vi "Array Test.vi"() -> ()   [LabVIEW 2016]
uses:
  Source/Shared Memory/Controls/file mode.ctl
  <vilib>/NI/Memory Manager/Classes/Pointer/Pointer.lvclass/Pointer.ctl
  <vilib>/NI/Memory Manager/Classes/Pointer/Write (1D DBL).vi
  <vilib>/NI/Memory Manager/Classes/Pointer/Read (1D DBL).vi
  <vilib>/NI/Memory Manager/Classes/Pointer/Write (1D Bool).vi
  <vilib>/NI/Memory Manager/Classes/Pointer/Read (1D Bool).vi
  <vilib>/NI/Memory Manager/Classes/Pointer/Write (No Check 1D DBL).vi
  <vilib>/NI/Memory Manager/Classes/Pointer/Check Null Pointer.vi
  <vilib>/NI/Memory Manager/Classes/Pointer/Check Subset (Power of 2).vi
  <vilib>/NI/Memory Manager/Classes/Pointer/Read (No Check 1D DBL).vi
  <vilib>/NI/Memory Manager/Classes/Pointer/Write (No Check 1D Bool).vi
  <vilib>/NI/Memory Manager/Classes/Pointer/Read (No Check 1D Bool).vi
  <vilib>/NI/Memory Manager/Classes/Pointer/Get Address.vi
  <vilib>/NI/Memory Manager/Classes/Pointer/Errors.vi
  <vilib>/NI/Memory Manager/Classes/Pointer/Null Pointer.vi
  <vilib>/NI/Memory Manager/Classes/Pointer/Out of Bounds.vi
  <vilib>/NI/Memory Manager/Classes/Pointer/Get Size.vi
  <vilib>/NI/Memory Manager/Classes/Pointer/Count to Size.vi
  <vilib>/NI/Memory Manager/Classes/Pointer/Create Error.vi
  <vilib>/NI/Memory Manager/VIs/Source.Write.String.vi
  <vilib>/NI/Memory Manager/Classes/Pointer/Write Pointer Size.vi
  <vilib>/NI/Memory Manager/VIs/Source.Write.Scalar.Base10.vi
  <vilib>/NI/Memory Manager/VIs/Source.Write.Scalar.Base10 (U64).vi
  <vilib>/NI/Memory Manager/VIs/New Error Cluster Constant.vi
  <vilib>/NI/Memory Manager/VIs/New Error Cluster Constant (512B).vi
  <vilib>/NI/Memory Manager/VIs/Error Cluster.Set Status.vi
  <vilib>/NI/Memory Manager/VIs/Error Cluster.Set Code.vi
  <vilib>/NI/Memory Manager/VIs/Error Cluster.Set VI Source.vi
  <vilib>/NI/Memory Manager/Constants/Constants.vi
  <vilib>/NI/Memory Manager/Constants/Library Name.vi
  <vilib>/NI/Memory Manager/Classes/Pointer/Get Error Info.vi
  Source/Shared Memory/Classes/Pointer/Shared Memory Pointer.lvclass
  C:/Program Files (x86)/National Instruments/LabVIEW 2016/vi.lib/NI/Memory Manager/Classes/Pointer/Pointer.lvclass
  Source/Shared Memory/Linux RT IPC.Shared Memory.lvlib
  Source/Shared Memory/Classes/Shared Memory/Shared Memory.lvclass
  <vilib>/NI/Memory Manager/Classes/Pointer/Pointer.lvclass
panel:
  out "error out":errorcluster
  in  "stop":bool
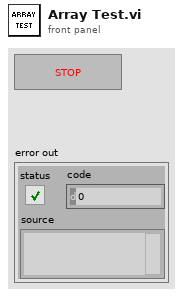
[diagram p1: front panel]
types:
  T1 = typedef "Linux RT IPC.Shared Memory.lvlib/file mode.ctl" = enum16{"open", "create/replace"}
  T2 = typedef "Linux RT IPC.Shared Memory.lvlib/reference.ctl" = refnum<data-value>
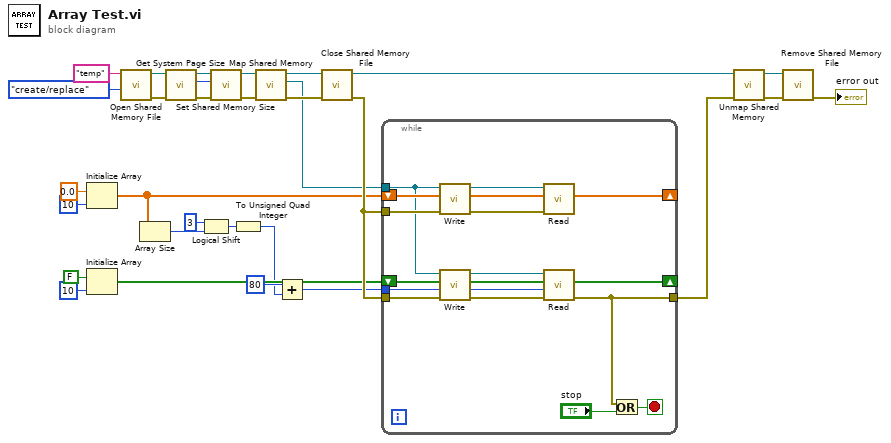
[diagram p0: block diagram]
diagram:
  n1 = Initialize Array(0.0 ("element"), 10 ("dimension size")) -> (w7:dbl[])
  n2 = Initialize Array(FALSE, 10 ("dimension size")) -> (w14:bool[])
  n3 = call "Open Shared Memory File.vi"("file mode (open)"=file_mode."create/replace" ("file mode (default: open)"), "shared memory name"="temp") -> ("error out"=w23:errorcluster, "shared memory out"=w24:T2)  [unwired: 8 in]
  n4 = Array Size(array=w7) -> (size(s)=w6:i32)
  n5 = call "Get System Page Size.vi"("error in (no error)"=w23, "shared memory in"=w24) -> ("error out"=w18:errorcluster, "page size (bytes)"=w19:u32, "shared memory out"=w22:T2)  [unwired: 7 in]
  n6 = Logical Shift(y=i16 3, x=w6) -> (x << y=w4:i32)
  n7 = call "Set Shared Memory Size.vi"("error in (no error)"=w18, "size (bytes)"=w19, "shared memory in"=w22) -> ("error out"=w20:errorcluster, "shared memory out"=w21:T2)  [unwired: 7 in]
  n8 = To Unsigned Quad Integer(1:w4) -> (0:w3:u64)
  n9 = call "Map Shared Memory.vi"("error in (no error)"=w20, "shared memory in"=w21) -> ("error out"=w16:errorcluster, "shared memory pointer"=w1:refnum<class "Shared Memory Pointer.lvclass">, "shared memory out"=w13:T2)  [unwired: 7 in]
  n10 = Add(x=u64 80 ("y"), y=w3) -> (x+y=w2:u64)
  n11 = call "Close Shared Memory File.vi"("error in (no error)"=w16, "shared memory in"=w13) -> ("error out"=w15:errorcluster, "shared memory out"=w12:T2)  [unwired: 8 in]
  n12 = while {
    shift-right: [w31] -> _
    shift-left: w7 -> [w39]
    shift-right: [w32] -> _
    shift-left: w14 -> [w46]
    tunnel: w2 -> [w45]
    tunnel: w15 -> [w44]
    tunnel: w15 -> [w43]
    tunnel: [w40] -> w10
    tunnel: w1 -> [w34]
    stop <- w41 stop-if-true
    n13 = call-poly <vilib>:"Write.vi"("error in (no error)"=w44, "buffer in"=w39, "Pointer in"=w34) -> ("error out"=w48:errorcluster, "buffer out"=w38:dbl[], "Pointer out"=w35:refnum<class "Shared Memory Pointer.lvclass">)  [unwired: 5 in, 1 out]
    n14 = call-poly <vilib>:"Write.vi"("error in (no error)"=w43, "offset (0)"=w45, "buffer in"=w46, "Pointer in"=w34) -> ("error out"=w47:errorcluster, "offset out"=w36:u64, "buffer out"=w37:bool[], "Pointer out"=w33:refnum<class "Shared Memory Pointer.lvclass">)  [unwired: 4 in]
    n15 = call-poly <vilib>:"Read.vi"("error in (no error)"=w48, "buffer in"=w38, "Pointer in"=w35) -> ("buffer out"=w31:dbl[])  [unwired: 5 in, 3 out]
    n16 = call-poly <vilib>:"Read.vi"("error in (no error)"=w47, "offset (0)"=w36, "buffer in"=w37, "Pointer in"=w33) -> ("error out"=w40:errorcluster, "buffer out"=w32:bool[])  [unwired: 4 in, 2 out]
    n17 = Or(x=w40, y="stop") -> (x .or. y?=w41:bool)
  }
  n18 = call "Unmap Shared Memory.vi"("error in (no error)"=w10, "shared memory in"=w12) -> ("error out"=w9:errorcluster, "shared memory out"=w11:T2)  [unwired: 8 in]
  n19 = call "Remove Shared Memory File.vi"("error in (no error)"=w9, "shared memory in"=w11) -> ("error out"=→"error out":errorcluster)  [unwired: 8 in, 1 out]
